vi "ReadPacket.vi"(10 "Reset":bool, 11 "Refnum in":refnum<k20>) -> (1 "ReadPacket":u8[](array[numeric]), 2 "Valid":bool, 3 "Complete":bool=TRUE)   [LabVIEW 2011]
uses:
  <vilib>/Utility/error.llb/Error Cluster From Error Code.vi
  <vilib>/rvi/errors/niLvFpgaAdjustHostInterfaceError.vi
  <vilib>/rvi/interface/nirviMethod/nirviMethod.xnode
  <vilib>/FPGAPlugInAG/Dynamic/niLvFpga_ReadFifo_Dynamic.vi
  <vilib>/rvi/errors/niLvFpgaMergeErrorWithErrorCode.vi
panel:
  in  "error in (no error)":errorcluster
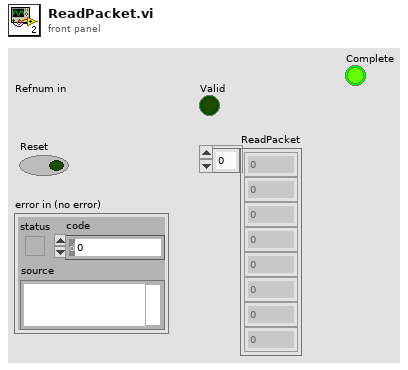
[diagram p1: front panel]
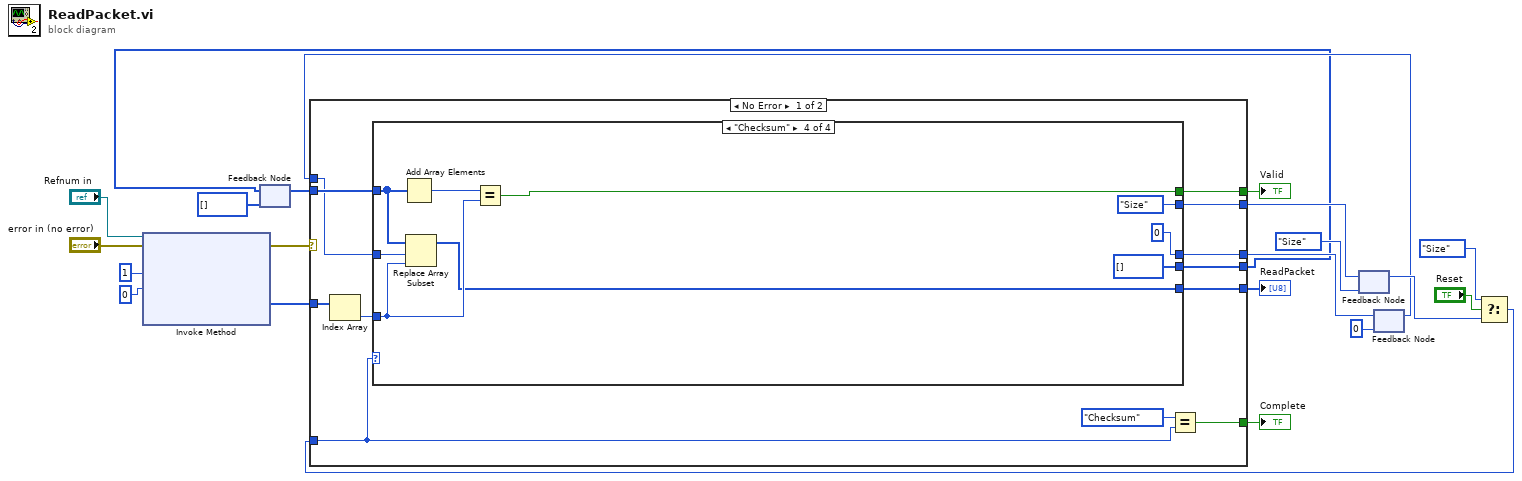
[diagram p0: block diagram]
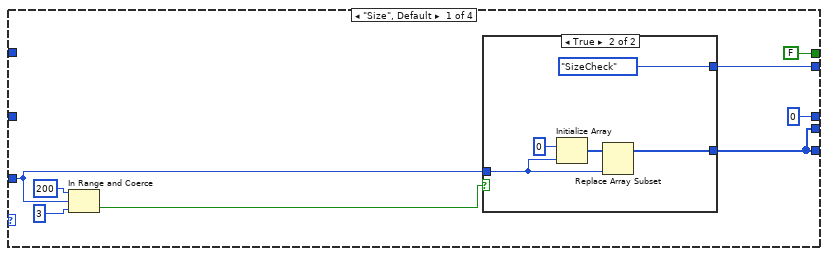
[diagram p2: hidden frame]
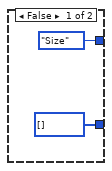
[diagram p3: hidden frame]
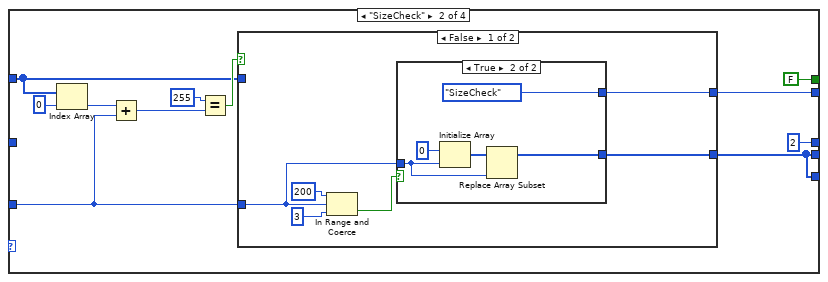
[diagram p4: hidden frame]
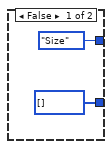
[diagram p5: hidden frame]
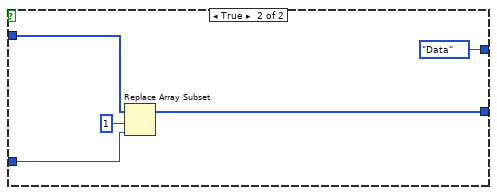
[diagram p6: hidden frame]
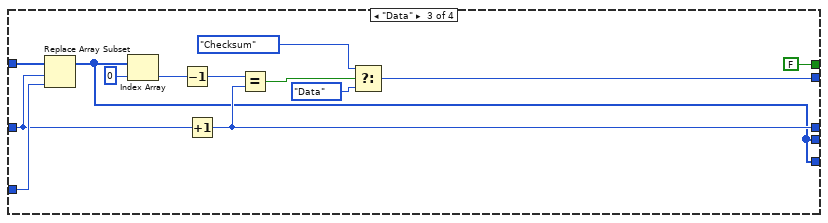
[diagram p7: hidden frame]
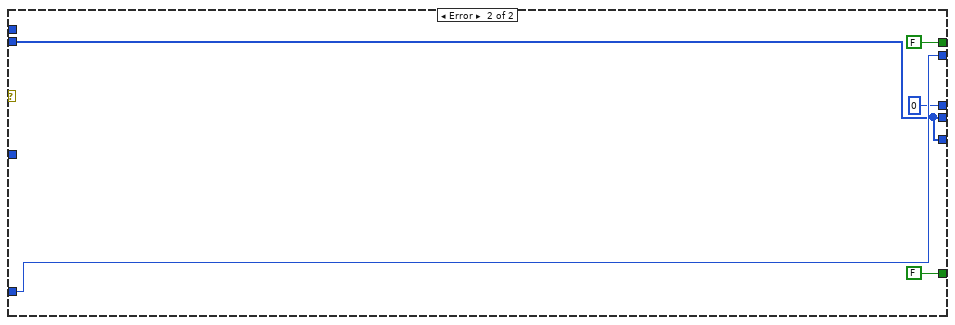
[diagram p8: hidden frame]
diagram:
  n1 = xnode "Invoke Method"("FPGA VI Reference In"="Refnum in", "error in"="error in (no error)", "Number of Elements"=u32 1, "Timeout (ms)"=0) -> ("error out"=w8:errorcluster, "Data"=w9:u8[])  [unwired: 2 out]
  n2 = feedback #1(u8[] []) -> (w12:u8[])
  n3 = feedback #2(enum16{"Size", "SizeCheck", "Data", "Checksum"}."Size") -> (w19:enum16{"Size", "SizeCheck", "Data", "Checksum"})
  n4 = feedback #3(0 ("index")) -> (w15:i32)
  n5 = Select(t=enum16{"Size", "SizeCheck", "Data", "Checksum"}."Size", s="Reset", f=w19) -> (s? t:f=w20:enum16{"Size", "SizeCheck", "Data", "Checksum"})
  n6 = case shown="No Error" w8 {
    tunnel: w9 -> [w33 _]
    tunnel: w20 -> [w24 w104]
    tunnel: [w31 w100] -> w11
    tunnel: w12 -> [w29 w100]
    tunnel: [w30 w104] -> w17
    tunnel: w15 -> [w28 _]
    tunnel: [w27 0 ("index")] -> w14
    tunnel: [w26 w100] -> w3
    tunnel: [w25 FALSE] -> w2
    tunnel: [w22 FALSE] -> w1
    frame No Error {
      n7 = Index Array(array=w33) -> (element=w32:u8)  [unwired: 1 in]
      n8 = case shown="\"Checksum\"" w24 {
        tunnel: w32 -> [w40 w53 w89 w93]
        tunnel: [w34 w49 w79 u8[] []] -> w31
        tunnel: [w41 w52 w83 enum16{"Size", "SizeCheck", "Data", "Checksum"}."Size"] -> w30
        tunnel: w29 -> [_ w54 w90 w95]
        tunnel: w28 -> [_ _ w82 w96]
        tunnel: [0 ("index") 2 ("index") w81 0 ("index")] -> w27
        tunnel: [w34 w49 w79 w92] -> w26
        tunnel: [FALSE FALSE FALSE w91] -> w25
        frame "Size", Default {
          n9 = In Range and Coerce(upper limit=u8 200, x=w40, lower limit=u8 3) -> (In Range?=w37:bool)  [unwired: 1 out]
          n10 = case shown="True" w37 {
            tunnel: w40 -> [_ w46]
            tunnel: [u8[] [] w45] -> w34
            tunnel: [enum16{"Size", "SizeCheck", "Data", "Checksum"}."Size" enum16{"Size", "SizeCheck", "Data", "Checksum"}."SizeCheck"] -> w41
            frame False {
            }
            frame True {
              n11 = Initialize Array(u8 0 ("element"), w46) -> (w47:u8[])
              n12 = Replace Array Subset(array=w47, new element=w46) -> (w45:u8[])  [unwired: 1 in]
            }
          }
        }
        frame "SizeCheck" {
          n13 = Index Array(array=w54, index=0) -> (element=w58:u8)
          n14 = Add(x=w58, y=w53) -> (x+y=w57:u8)
          n15 = Equal?(x=u8 255, y=w57) -> (x = y?=w55:bool)
          n16 = case shown="False" w55 {
            tunnel: w54 -> [_ w77]
            tunnel: w53 -> [w62 w75]
            tunnel: [w61 w74] -> w49
            tunnel: [w60 enum16{"Size", "SizeCheck", "Data", "Checksum"}."Data"] -> w52
            frame False {
              n17 = In Range and Coerce(upper limit=u8 200, x=w62, lower limit=u8 3) -> (In Range?=w63:bool)  [unwired: 1 out]
              n18 = case shown="True" w63 {
                tunnel: w62 -> [_ w70]
                tunnel: [u8[] [] w69] -> w61
                tunnel: [enum16{"Size", "SizeCheck", "Data", "Checksum"}."Size" enum16{"Size", "SizeCheck", "Data", "Checksum"}."SizeCheck"] -> w60
                frame False {
                }
                frame True {
                  n19 = Initialize Array(u8 0 ("element"), w70) -> (w71:u8[])
                  n20 = Replace Array Subset(array=w71, new element=w70) -> (w69:u8[])  [unwired: 1 in]
                }
              }
            }
            frame True {
              n21 = Replace Array Subset(array=w77, new element=w75, index=1) -> (w74:u8[])
            }
          }
        }
        frame "Data" {
          n22 = Replace Array Subset(array=w90, new element=w89, index=w82) -> (w79:u8[])
          n23 = Index Array(array=w79, index=0) -> (element=w87:u8)
          n24 = Decrement(x=w87) -> (x-1=w80:u8)
          n25 = Increment(x=w82) -> (x+1=w81:i32)
          n26 = Equal?(x=w80, y=w81) -> (x = y?=w86:bool)
          n27 = Select(t=enum16{"Size", "SizeCheck", "Data", "Checksum"}."Checksum", s=w86, f=enum16{"Size", "SizeCheck", "Data", "Checksum"}."Data") -> (s? t:f=w83:enum16{"Size", "SizeCheck", "Data", "Checksum"})
        }
        frame "Checksum" {
          n28 = Add Array Elements(numeric array=w95) -> (sum=w94:u8)
          n29 = Replace Array Subset(array=w95, new element=w93, index=w96) -> (w92:u8[])
          n30 = Equal?(x=w94, y=w93) -> (x = y?=w91:bool)
        }
      }
      n31 = Equal?(x=enum16{"Size", "SizeCheck", "Data", "Checksum"}."Checksum", y=w24) -> (x = y?=w22:bool)
    }
    frame Error {
    }
  }
  "ReadPacket" <- w3
  "Valid" <- w2
  "Complete" <- w1
  n32 = feedback-in #1(w11) -> ()
  n33 = feedback-in #2(w17) -> ()
  n34 = feedback-in #3(w14) -> ()
